vi "Simulation Noninteractive Run.vi"(11 "simulation configuration":T2={"maxTime"=inf, "enableVisualization"=TRUE, "statechart"=path "Simulation Statechart.vi", "environment"=path "Environment - Navigation and Hill Climb 1.xml", "record"=path "Simulation Record.xml", "autograde?"=TRUE, "interactive?"=FALSE, "feedback mode"=enum."debug navigation"}) -> (0 "error out":errorcluster, 3 "record":T1={"configuration"={"maxTime"=5.0, "enableVisualization"=TRUE, "statechart"=path "iRobot Navigation State Machine.vi", "environment"=path "iRobot Navigation State Machine.vi", "record"=path "Simulation Record.xml", "autograde?"=TRUE, "interactive?"=FALSE, "feedback mode"=enum."debug navigation"}, "trace"=[], "environment MD5"="", "statechart MD5"="", "record timestamp"=""} {"trace"."sensors"."iRobot Sensors"."Infrared" format="%02x"; "trace"."sensors"."accelerometer"."z axis (g)" format="%.3f"; "trace"."sensors"."accelerometer"."y axis (g)" format="%.3f"; "trace"."sensors"."accelerometer"."x axis (g)" format="%.3f"})   [LabVIEW 2013]
uses:
  CyberSim interface/Simulation Configuration.ctl
  autograder/feedbackMode.ctl
  Simulation Record.ctl
  Simulation Trace Element.ctl
  shared/Sensors.ctl
  iRobot/Sensor/Accelerometer.ctl
  iRobot/Sensor/Sensor Group 6.ctl
  iRobot/Sensor/Bumps + Wheel Drops.ctl
  iRobot/Sensor/Buttons.ctl
  iRobot/Sensor/Charging State.ctl
  iRobot/Sensor/Charging Sources Available.ctl
  iRobot/Sensor/OI Mode.ctl
  iRobot/Sensor/Cargo Bay Digital Inputs.ctl
  iRobot/Sensor/Low-Side Driver + Wheel Overcurrent.ctl
  Simulated iRobot Position.ctl
  Simulated iRobot Orientation.ctl
  Simulation Call Statechart Operation.ctl
panel:
  # "Electrical: charging, battery, OI mode"
  # "Sensors: bump, cliff, button, wheel drop, wall, virtual wall"
  # "Motion: distance, angle, requested velocity"
  # "Cargo Bay: I/O, overcurrent, infrared"
  # "Song"
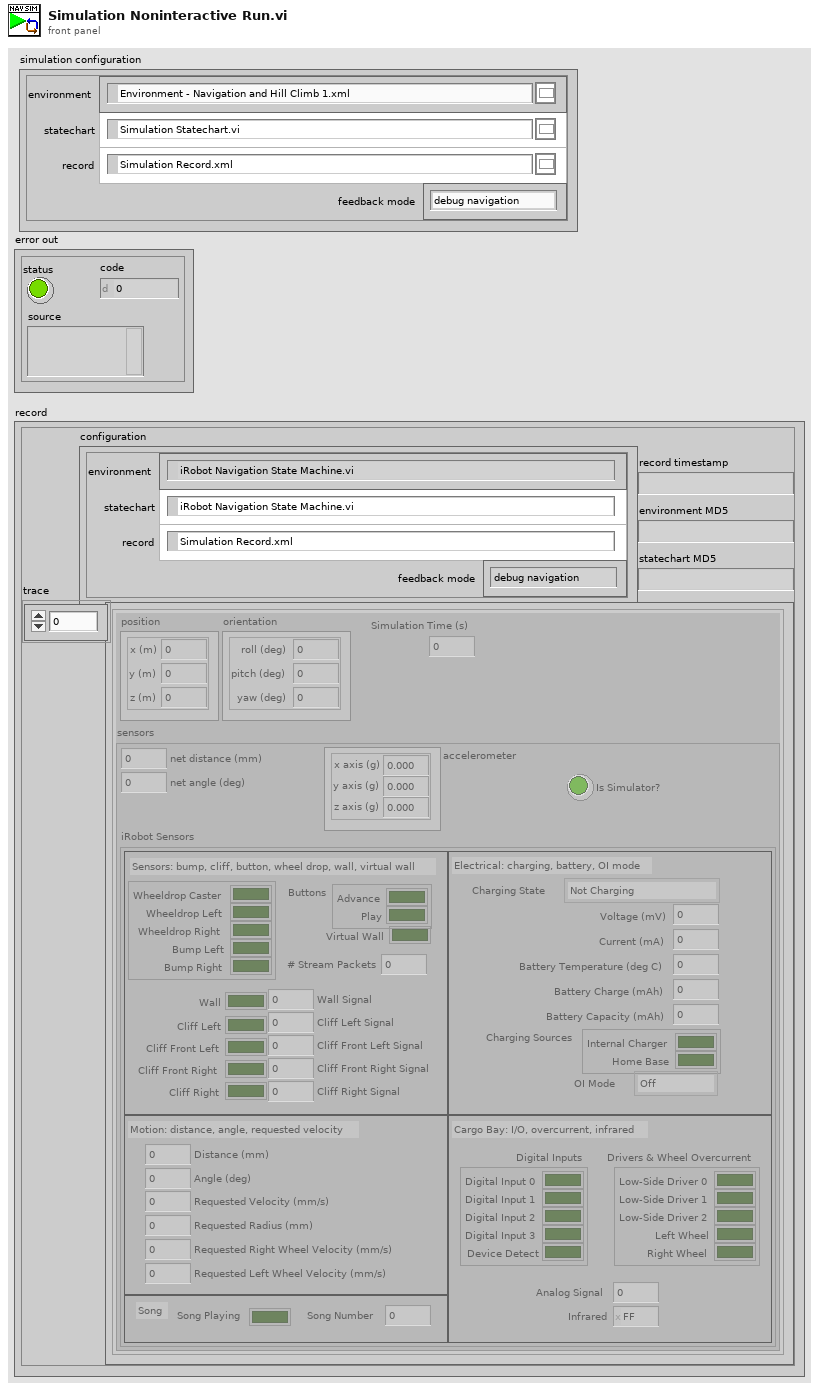
[diagram p1: front panel]
types:
  T1 = typedef "Simulation Record.ctl" = cluster{"configuration":T2, "trace":T4[], "environment MD5":string, "statechart MD5":string, "record timestamp":string}
  T2 = typedef "Simulation Configuration.ctl" = cluster{"maxTime":sgl, "enableVisualization":bool, "statechart":path, "environment":path, "record":path, "autograde?":bool, "interactive?":bool, "feedback mode":T3}
  T3 = typedef "feedbackMode.ctl" = enum32{"debug navigation", "debug hill climb", "autograde navigation", "autograde hill climb"}
  T4 = typedef "Simulation Trace Element.ctl" = cluster{"sensors":T5, "position":T15, "orientation":T16, "Simulation Time (s)":sgl}
  T5 = typedef "Sensors.ctl" = cluster{"net distance (mm)":i32, "net angle (deg)":i32, "accelerometer":T6, "iRobot Sensors":T7, "Is Simulator?":bool}
  T6 = typedef "Accelerometer.ctl" = cluster{"x axis (g)":dbl, "y axis (g)":dbl, "z axis (g)":dbl}
  T7 = typedef "Sensor Group 6.ctl" = cluster{"Bumps + Wheel Drops":T8, "Wall":bool, "Cliff Left":bool, "Cliff Front Left":bool, "Cliff Front Right":bool, "Cliff Right":bool, "Wall Signal":u16, "Cliff Left Signal":u16, "Cliff Front Left Signal":u16, "Cliff Front Right Signal":u16, "Cliff Right Signal":u16, "Buttons":T9, "Virtual Wall":bool, "# Stream Packets":u8, "Requested Velocity (mm/s)":i16, "Requested Radius (mm)":i16, "Requested Right Wheel Velocity (mm/s)":i16, "Requested Left Wheel Velocity (mm/s)":i16, "Distance (mm)":i32, "Angle (deg)":i32, "Song Playing":bool, "Song Number":u8, "Charging State":T10, "Voltage (mV)":u16, "Current (mA)":i16, "Battery Temperature (deg C)":i8, "Battery Charge (mAh)":u16, "Battery Capacity (mAh)":u16, "Charging Sources":T11, "OI Mode":T12, "Digital Inputs":T13, "Drivers & Wheel Overcurrent":T14, "Analog Signal":u16, "Infrared":u8}
  T8 = typedef "Bumps + Wheel Drops.ctl" = cluster{"Wheeldrop Caster":bool, "Wheeldrop Left":bool, "Wheeldrop Right":bool, "Bump Left":bool, "Bump Right":bool}
  T9 = typedef "Buttons.ctl" = cluster{"Advance":bool, "Play":bool}
  T10 = typedef "Charging State.ctl" = enum16{"Not Charging", "Reconditioning Charging", "Full Charging", "Trickle Charging", "Waiting", "Charging Fault Condition"}
  T11 = typedef "Charging Sources Available.ctl" = cluster{"Internal Charger":bool, "Home Base":bool}
  T12 = typedef "OI Mode.ctl" = enum16{"Off", "Passive", "Safe", "Full"}
  T13 = typedef "Cargo Bay Digital Inputs.ctl" = cluster{"Digital Input 0":bool, "Digital Input 1":bool, "Digital Input 2":bool, "Digital Input 3":bool, "Device Detect":bool}
  T14 = typedef "Low-Side Driver + Wheel Overcurrent.ctl" = cluster{"Low-Side Driver 0":bool, "Low-Side Driver 1":bool, "Low-Side Driver 2":bool, "Left Wheel":bool, "Right Wheel":bool}
  T15 = typedef "Simulated iRobot Position.ctl" = cluster{"x (m)":sgl, "y (m)":sgl, "z (m)":sgl}
  T16 = typedef "Simulated iRobot Orientation.ctl" = cluster{"roll (deg)":sgl, "pitch (deg)":sgl, "yaw (deg)":sgl}
  T17 = typedef "Simulation Call Statechart Operation.ctl" = enum16{"Initialize", "Call Statechart", "Finalize"}
  T18 = typedef "Simulator.ctl" = cluster{"configuration":T2, "Bump Sensors":refnum<k20>[], "Distance Sensors":refnum<k20>[], "Accelerometer":refnum<k20>, "Wall Sensor":refnum<k20>, "Statechart\ndisplay":refnum<vi>, "Body":refnum<k20>, "Left Motor":refnum<class "DC Motor Controller.lvclass">, "Right Motor":refnum<class "DC Motor Controller.lvclass">, "first step?":bool}
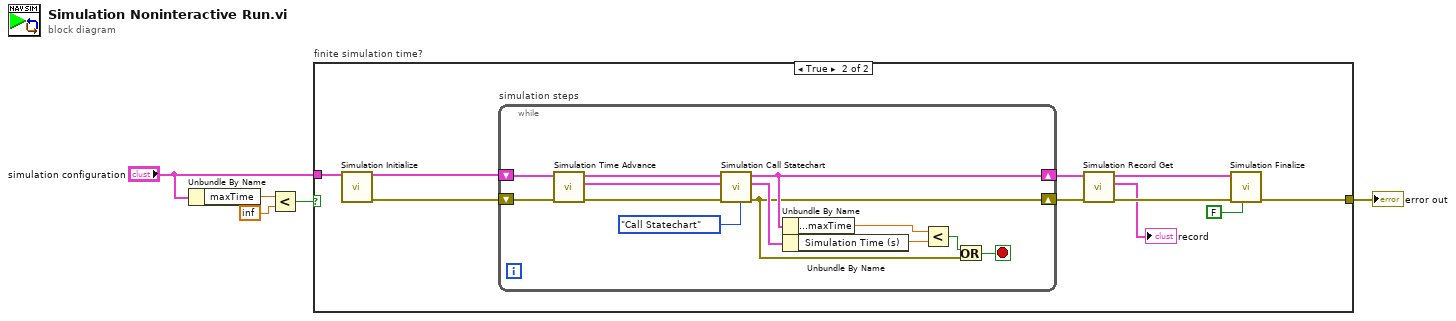
[diagram p0: block diagram]
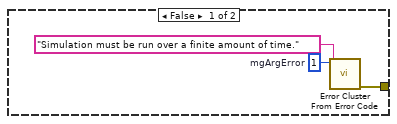
[diagram p2: hidden frame]
diagram:
  n1 = Unbundle By Name("simulation configuration") -> ("maxTime"=w3:sgl)
  n2 = Less?(x=w3, y=sgl inf) -> (x < y?=w1:bool)
  n3 = case "finite simulation time?" shown="True" w1 {
    tunnel: [w8 w16] -> w5
    tunnel: "simulation configuration" -> [_ w15]
    frame False {
      w7 = 1  # mgArgError
      n4 = call <vilib>:"Error Cluster From Error Code.vi"("error message (\"\")"="Simulation must be run over a finite amount of time." ("error message (\"\")"), "error code (0)"=w7) -> ("error out"=w8:errorcluster)  [unwired: 7 in]
    }
    frame True {
      n5 = call "Simulation Initialize.vi"("simulation configuration"=w15) -> ("simulator"=w18:T18, "Error Out"=w17:errorcluster)  [unwired: 13 in]
      n6 = while "simulation steps" {
        shift-right: [w20] -> w14
        shift-left: w18 -> [w27]
        shift-right: [w19] -> w13
        shift-left: w17 -> [w26]
        stop <- w21 stop-if-true
        n7 = call "Simulation Time Advance.vi"("error in (no error)"=w26, "simulator"=w27) -> ("error out"=w29:errorcluster, "sensors"=w30:T5, "simulator"=w31:T18)  [unwired: 7 in]
        n8 = call "Simulation Call Statechart.vi"("operation"=Simulation_Call_Statechart_Operation."Call Statechart", "error in"=w29, "sensors"=w30, "simulator"=w31) -> ("error out"=w19:errorcluster, "trace element"=w23:T4, "simulator"=w20:T18)  [unwired: 5 in]
        n9 = Unbundle By Name(w20) -> ("configuration.maxTime"=w25:sgl)
        n10 = Unbundle By Name(w23) -> ("Simulation Time (s)"=w24:sgl)
        n11 = Less?(x=w25, y=w24) -> (x < y?=w22:bool)
        n12 = Or(x=w22, y=w19) -> (x .or. y?=w21:bool)
      }
      n13 = call "Simulation Record Get.vi"("Error In"=w13, "simulator"=w14) -> ("Error Out"=w11:errorcluster, "record"=→"record":T1, "simulator"=w12:T18)  [unwired: 7 in]
      n14 = call "Simulation Finalize.vi"("terminated by user?"=FALSE, "error in (no error)"=w11, "simulator"=w12) -> ("error out"=w16:errorcluster)  [unwired: 7 in, 1 out]
    }
  }
  "error out" <- w5
